vi "Write Outputs Zero.vi"(8 "error in (no error)":errorcluster, 11 "Analog Writer in":refnum<class "Analog Writer.lvclass">) -> (0 "error out":errorcluster, 3 "Analog Writer out":refnum<class "Analog Writer.lvclass">)   [LabVIEW 2024, in "DAQmx Actor.lvlib" / "Analog Writer.lvclass"]
uses:
  Analog Writer.lvclass
  Analog Writer.lvclass/Analog Writer.ctl
  <resource>/objmgr/daqmx.rc
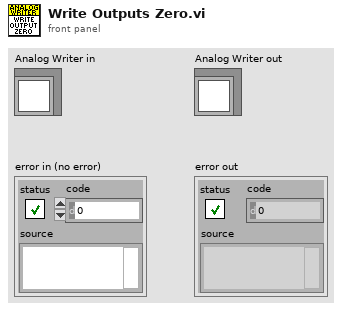
[diagram p1: front panel]
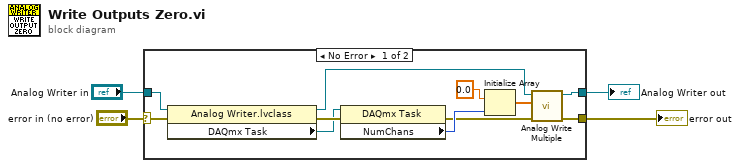
[diagram p0: block diagram]
diagram:
  n1 = case shown="No Error" "error in (no error)" {
    selector: "error in (no error)" -> [w5 w17]
    tunnel: [w6 w17] -> w3
    tunnel: [w7 w16] -> w1
    tunnel: "Analog Writer in" -> [w9 w16]
    frame No Error {
      n2 = property class="Analog Writer.lvclass"(reference=w9, error in=w5) -> (reference out=w8:refnum<class "Analog Writer.lvclass">, error out=w15:errorcluster, "DAQmx Task"=w14:refnum<k21>)
      n3 = property class="DAQmx Task"(reference=w14, error in=w15) -> (error out=w10:errorcluster, "NumChans"=w13:u32)  [unwired: 1 out]
      n4 = Initialize Array(0.0, w13) -> (w11:dbl[])
      n5 = call-dynamic "Analog Write Multiple.vi"("error in (no error)"=w10, "Analog Data"=w11, "Analog Writer in"=w8) -> ("error out"=w6:errorcluster, "Analog Writer out"=w7:refnum<class "Analog Writer.lvclass">)  [unwired: 7 in]
    }
    frame Error {
    }
  }
  "error out" <- w3
  "Analog Writer out" <- w1
